vi "Delacor_lib_QMH_Enqueue Message (Single).vi"(6 "Priority Message? (F)":bool, 8 "error in":errorcluster, 9 "Message Data":variant, 10 "Message":string, 11 "Message Queue in":refnum<class "RQMHMessageQueue.lvclass">) -> (0 "error out":errorcluster, 3 "Message Queue out":refnum<class "RQMHMessageQueue.lvclass">)   [LabVIEW 2024, in "RQMHMessageQueue.lvclass"]
doc: "For a regular message, enqueue the message. For a priority message, enqueue it at the front of the queue.\nThis is an instance of the polymorphic VI: \"Enqueue Message (poly).vi\"\n____\nDQMH Framework: Palette 7.1.0.1503\nCopyright (c) 2025, DQMH Consortium"
uses:
  RQMHMessageQueue.lvclass
  RQMHMessageQueue.lvclass/RQMHMessageQueue.ctl
  Delacor_lib_QMH_Message--cluster.ctl
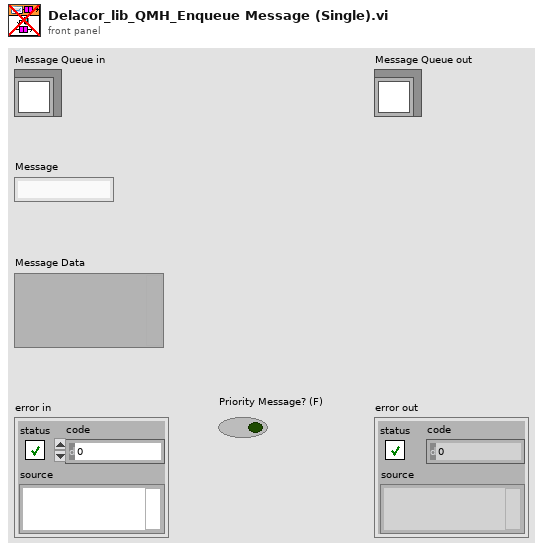
[diagram p1: front panel]
types:
  T1 = typedef "RQMHMessageQueue.lvclass/Delacor_lib_QMH_Message--cluster.ctl" = cluster{"Message":string, "Message Data":variant}
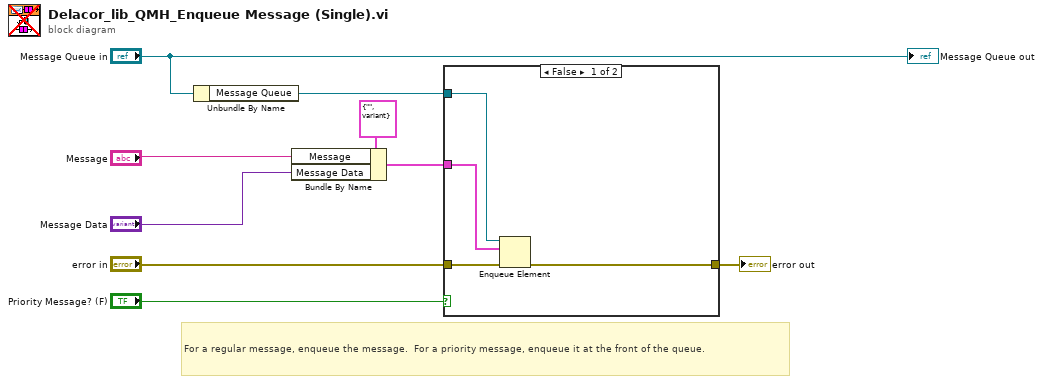
[diagram p0: block diagram]
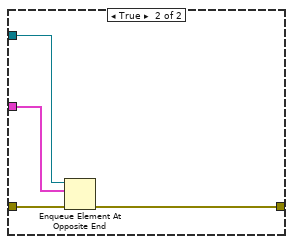
[diagram p2: hidden frame]
diagram:
  # "For a regular message, enqueue the message.  For a priority message, enqueue it at the front of the queue."
  n1 = Unbundle By Name("Message Queue in") -> ("Message Queue"=w2:refnum<queue>)
  n2 = Bundle By Name(cluster=T1 {"Message"="", "Message Data"=variant} ("Message Cluster"), "Message"="Message", "Message Data"="Message Data") -> (w3:T1)
  n3 = case shown="False" "Priority Message? (F)" {
    tunnel: "error in" -> [w13 w17]
    tunnel: [w12 w16] -> w8
    tunnel: w2 -> [w10 w15]
    tunnel: w3 -> [w11 w14]
    frame False {
      n4 = Enqueue Element(queue=w10, element=w11, error in (no error)=w13) -> (error out=w12:errorcluster)  [unwired: 1 in, 2 out]
    }
    frame True {
      n5 = Enqueue Element At Opposite End(queue=w15, element=w14, error in (no error)=w17) -> (error out=w16:errorcluster)  [unwired: 1 in, 2 out]
    }
  }
  "error out" <- w8
  "Message Queue out" <- "Message Queue in"
